vi "Lab02_BradsWay.vi"() -> ()   [LabVIEW 2022 SP3]
panel:
  out "Array":i32[](array[numeric])
  out "Numeric":i32
  in  "Go":bool
  in  "Stop":bool
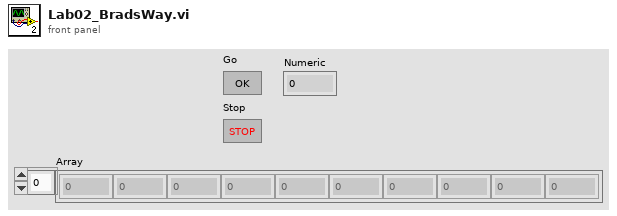
[diagram p1: front panel]
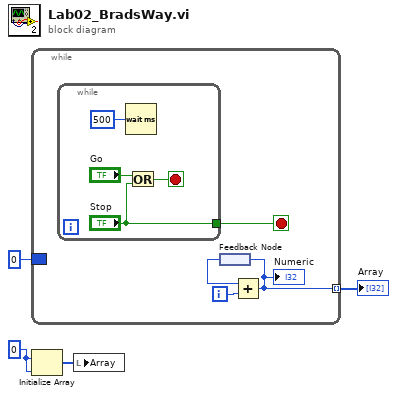
[diagram p0: block diagram]
diagram:
  w2 = 0 ("dimension size")
  n1 = while {
    tunnel: [w7] -> w3 mode=indexing
    border: 0 -> [_]
    i -> [w5]
    stop <- w6 stop-if-true
    n2 = while {
      tunnel: ["Stop"] -> w6
      stop <- w12 stop-if-true
      n3 = Wait (ms)(milliseconds to wait=u32 500) -> ()  [unwired: 1 out]
      n4 = Or(x="Go", y="Stop") -> (x .or. y?=w12:bool)
    }
    n5 = feedback #1() -> (w8:i32)
    n6 = Add(x=w8, y=w5) -> (x+y=w7:i32)
    "Numeric" <- w7
    n7 = feedback-in #1(w7) -> ()
  }
  "Array" <- w3
  n8 = Initialize Array(w2, w2) -> (w1:i32[])
  n9 = local write "Array"(w1) -> ()
